vi "Write GroupName.vi"(8 "error in":errorcluster, 10 "groupName":string, 11 "group in":refnum<class "group node.lvclass">) -> (0 "error out":errorcluster, 3 "group out":refnum<class "group node.lvclass">)   [LabVIEW 2013, in "group node.lvclass"]
uses:
  group node.lvclass
  group node.lvclass/group node.ctl
  Configuration Framework/serializable configuration/set metadata property.vi
  group configuration/group configuration.lvclass
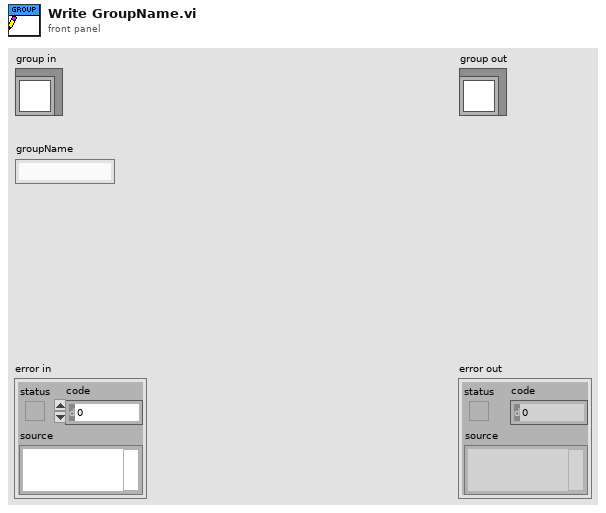
[diagram p1: front panel]
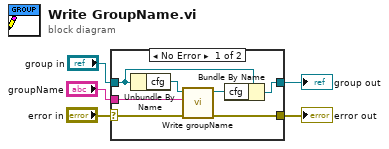
[diagram p0: block diagram]
diagram:
  n1 = case shown="No Error" "error in" {
    selector: "error in" -> [w7 w13]
    tunnel: [w10 w13] -> w4
    tunnel: [w12 w14] -> w2
    tunnel: "group in" -> [w11 w14]
    tunnel: "groupName" -> [w6 _]
    frame No Error {
      n2 = Unbundle By Name(w11) -> ("cfg"=w8:refnum<class "group configuration.lvclass">)
      n3 = call "Write groupName.vi"("error in (no error)"=w7, "groupName"=w6, "group configuration in"=w8) -> ("error out"=w10:errorcluster, "group configuration out"=w9:refnum<class "group configuration.lvclass">)  [unwired: 7 in]
      n4 = Bundle By Name(cluster=w11, "cfg"=w9) -> (w12:refnum<class "group node.lvclass">)
    }
    frame Error {
    }
  }
  "error out" <- w4
  "group out" <- w2
